vi "FOCUS_V42_H37.vi"(9 "X-pixels":sgl=256.0, 11 "Run":bool) -> (0 "Retrace pixels":sgl, 10 "Pixel Clock (Hz)":sgl)   [LabVIEW 2010] (continued)
                            n2198 = To Unsigned Byte Integer(number=w3929) -> (unsigned 8bit integer=w3921:u8[])
                            n2199 = Add(x=w3896, y=w3900) -> (x+y=w3905:sgl[])
                            n2200 = To Unsigned Byte Integer(number=w3905) -> (unsigned 8bit integer=w3893:u8[])
                          }
                        }
                      }
                    }
                    n2201 = case shown="True" "Overlay Images" {
                      tunnel: w3666 -> [w4140 w4159]
                      tunnel: [w4140 w4142] -> w3813
                      tunnel: w3665 -> [w4139 w4161]
                      tunnel: [w4139 _] -> w3814
                      frame False {
                      }
                      frame True {
                        n2202 = To Word Integer(number=w4159) -> (16bit integer=w4160:i16[])
                        n2203 = Subtract(x=w4160, y=w4161) -> (x-y=w4141:i16[])
                        n2204 = Add(x=w4160, y=w4161) -> (x+y=w4155:i16[])
                        n2205 = Increment(x=w4155) -> (x+1=w4165:i16[])
                        n2206 = Divide(x=w4141, y=w4165) -> (x/y=w4164:dbl[])
                        n2207 = Absolute Value(x=w4141) -> (abs(x)=w4157:i16[])
                        n2208 = Multiply(x=w4164, y=u8 2) -> (x*y=w4162:dbl[])
                        n2209 = Round To Nearest(number=w4162) -> (nearest integer value=w4148:dbl[])
                        n2210 = Divide(x=w4157, y=2.0) -> (x/y=w4154:dbl[])
                        n2211 = Divide(x=w4155, y=2.0) -> (x/y=w4153:dbl[])
                        n2212 = Add(x=w4154, y=w4153) -> (x+y=w4151:dbl[])
                        n2213 = Divide(x=w4151, y=5.0) -> (x/y=w4150:dbl[])
                        n2214 = Round To Nearest(number=w4150) -> (nearest integer value=w4149:dbl[])
                        n2215 = Multiply(x=5.0 ("y"), y=w4149) -> (x*y=w4147:dbl[])
                        n2216 = Add(x=w4148, y=w4147) -> (x+y=w4146:dbl[])
                        n2217 = Subtract(x=w4146, y=2.0) -> (x-y=w4143:dbl[])
                        n2218 = To Unsigned Byte Integer(number=w4143) -> (unsigned 8bit integer=w4142:u8[])
                      }
                    }
                    n2219 = Greater Or Equal?(x=w3724, y=w3723) -> (x >= y?=w3658:bool)
                    n2220 = Sign(1:w3762) -> (0:w3761:i32)
                    n2221 = local write "Scan Backlock"(w3712) -> ()
                    n2222 = case shown="-1" w3761 {
                      tunnel: "Zoom" -> [_ w3966 w3971]
                      frame 0, Default {
                      }
                      frame 1 {
                        n2223 = Multiply(x=w3966, y=sgl 1.25) -> (x*y=w3964:sgl)
                        n2224 = local write "Zoom"(w3964) -> ()
                      }
                      frame -1 {
                        n2225 = Multiply(x=w3971, y=sgl 0.8) -> (x*y=w3967:sgl)
                        n2226 = Greater Or Equal?(x=w3967, y=sgl 0.28) -> (x >= y?=w3969:bool)
                        n2227 = case shown="True" w3969 {
                          tunnel: w3967 -> [_ w3972]
                          frame False {
                          }
                          frame True {
                            n2228 = local write "Zoom"(w3972) -> ()
                          }
                        }
                      }
                    }
                    n2229 = Not(x=w3681) -> (.not. x?=→"On?":bool)
                    n2230 = case shown="True" w3658 {
                      tunnel: w3770 -> [w3976 w4005]
                      tunnel: [w3976 w4004] -> w3769
                      tunnel: w3768 -> [w3977 w3983]
                      tunnel: [w3977 w3991] -> w3767
                      tunnel: w3719 -> [w3974 w3988]
                      tunnel: w3720 -> [w3975 w3985]
                      tunnel: [w3975 w3986] -> w3722
                      tunnel: [w3974 w3989] -> w3721
                      tunnel: [w3973 w3982] -> w3718
                      tunnel: w3717 -> [w3973 w3981]
                      tunnel: "scattering length [µm]" -> [_ w3978]
                      frame False {
                      }
                      frame True {
                        n2231 = local read "Sutter scale z"() -> (w3979:sgl)
                        n2232 = call "VISA MP-285 Get Z Position.vi"("Input: Duty Cluster"=w4005) -> ("Output: Z axis (microns)"=w4003:sgl, "Output: Duty Cluster"=w4004:T18, "error?"=w3982:bool)
                        n2233 = Multiply(x=w3979, y=w4003) -> (x*y=w3991:sgl)
                        n2234 = Equal?(x=TRUE, y="GetFirst") -> (x = y?=w3995:bool)
                        n2235 = Not Equal?(x="GetFirst", y=w3985) -> (x != y?=w3994:bool)
                        n2236 = Equal?(x=TRUE, y="GetLast") -> (x = y?=w3997:bool)
                        n2237 = Not Equal?(x="GetLast", y=w3988) -> (x != y?=w3999:bool)
                        n2238 = Subtract(x=w3991, y=w3983) -> (x-y=w4000:sgl)
                        n2239 = And(x=w3982, y=w3981) -> (x .and. y?=w3980:bool)
                        n2240 = Not Equal To 0?(x=w4000) -> (x != 0?=w4002:bool)
                        n2241 = Compound Arithmetic op=AND(w3995, w3994, w3980) -> (w3993:bool)
                        n2242 = Compound Arithmetic op=AND(w3980, w3997, w3999) -> (w3992:bool)
                        n2243 = Compound Arithmetic op=AND("IntensityAutomatic", w4002, w3980) -> (w3984:bool)
                        n2244 = case shown="True" w3993 {
                          tunnel: w3991 -> [_ w4008]
                          tunnel: "GetFirst" -> [_ w4007]
                          tunnel: [w4006 w4007] -> w3986
                          tunnel: w3985 -> [w4006 _]
                          frame False {
                          }
                          frame True {
                            "FirstPosition" <- w4008
                          }
                        }
                        n2245 = case shown="True" w3992 {
                          tunnel: w3991 -> [_ w4011]
                          tunnel: "GetLast" -> [_ w4010]
                          tunnel: [w4009 w4010] -> w3989
                          tunnel: w3988 -> [w4009 _]
                          frame False {
                          }
                          frame True {
                            "LastPosition" <- w4011
                          }
                        }
                        n2246 = case shown="True" w3984 {
                          tunnel: w4000 -> [_ w4015]
                          tunnel: w3991 -> [_ w4014]
                          tunnel: [w4012 w4014] -> _
                          tunnel: w3983 -> [w4012 _]
                          tunnel: w3978 -> [_ w4013]
                          frame False {
                          }
                          frame True {
                            n2247 = Divide(x=w4015, y=w4013) -> (x/y=w4022:sgl)
                            n2248 = local read "Intensity"() -> (w4020:sgl)
                            n2249 = Exponential(1:w4022) -> (0:w4021:sgl)
                            n2250 = local read "IntensityScaleMax"() -> (w4016:sgl)
                            n2251 = Multiply(x=w4020, y=w4021) -> (x*y=w4018:sgl)
                            n2252 = In Range and Coerce(upper limit=sgl 0.0, x=w4018, lower limit=w4016) -> (coerced(x)=w4017:sgl)  [unwired: 1 out]
                            n2253 = local write "Intensity"(w4017) -> ()
                          }
                        }
                      }
                    }
                    n2254 = Greater Or Equal?(x=w3812, y="Image Update [ms]") -> (x >= y?=w3810:bool)
                    n2255 = Greater Or Equal?(x=w3726, y=w3723) -> (x >= y?=w3654:bool)
                    n2256 = Replace Array Subset(array=w3771, new element=w3813, index (col)=w3726) -> (w3808:u8[][])  [unwired: 1 in]
                    n2257 = Replace Array Subset(array=w3778, new element=w3814, index (col)=w3726) -> (w3807:u8[][])  [unwired: 1 in]
                    n2258 = case shown="True" w3810 {
                      tunnel: [w4135 w4138] -> w3809
                      tunnel: w3795 -> [w4135 _]
                      tunnel: w3808 -> [_ w4137]
                      tunnel: w3807 -> [_ w4136]
                      frame False {
                      }
                      frame True {
                        n2259 = local write "Image 1"(w4137) -> ()
                        n2260 = local write "Image 2"(w4136) -> ()
                        n2261 = Tick Count (ms)() -> (millisecond timer value=w4138:u32)
                      }
                    }
                    n2262 = Unbundle By Name(w3743) -> ("status"=w3738:bool)
                    n2263 = case shown="False" w3654 {
                      tunnel: [w4038 i16 0] -> w3800
                      tunnel: w3726 -> [w4039 _]
                      frame False {
                        n2264 = Increment(x=w4039) -> (x+1=w4038:i16)
                      }
                      frame True {
                      }
                    }
                    n2265 = Unbundle By Name(w3742) -> ("status"=w3673:bool)
                    n2266 = case shown="False" w3658 {
                      tunnel: [w3957 i16 0] -> w3725
                      tunnel: w3724 -> [w3958 _]
                      frame False {
                        n2267 = Increment(x=w3958) -> (x+1=w3957:i16)
                      }
                      frame True {
                      }
                    }
                    n2268 = case shown="True" w3655 {
                      tunnel: w3666 -> [w3820 w3823]
                      tunnel: w3665 -> [w3817 w3822]
                      tunnel: w3664 -> [w3819 _]
                      tunnel: [w3818 w3821] -> w3661
                      frame True {
                        n2269 = Interleave 1D Arrays(w3817, w3820, w3819) -> (w3818:u8[])
                      }
                      frame False {
                        n2270 = Interleave 1D Arrays(w3823, w3822) -> (w3821:u8[])
                      }
                    }
                    n2271 = case shown="True" w3654 {
                      tunnel: w3663 -> [w3833 w3841]
                      tunnel: w3662 -> [w3832 w3840]
                      tunnel: w3661 -> [w3831 w3839]
                      tunnel: [w3830 w3838] -> w3660
                      tunnel: [w3829 w3837] -> w3659
                      frame True {
                        n2272 = Set File Position(offset (in bytes) (0)=768 ("pos offset (0)"), refnum=w3833, from (0:start)=enum16{"start", "end", "current"}."start" ("pos mode (0:2)"), error in=w3832) -> (refnum out=w3826:refnum<file>, error out=w3825:errorcluster)
                        n2273 = Write to Binary File(file (use dialog)=w3826, data=w3831, error in=w3825, 5:FALSE ("prepend array or string size? (T)")) -> (refnum out=w3830:refnum<file>, error out=w3829:errorcluster)  [unwired: 2 in, 1 out]
                      }
                      frame False {
                        n2274 = Set File Position(refnum=w3841, from (0:start)=enum16{"start", "end", "current"}."current" ("pos mode (0:2)"), error in=w3840) -> (refnum out=w3836:refnum<file>, error out=w3835:errorcluster)  [unwired: 1 in]
                        n2275 = Write to Binary File(file (use dialog)=w3836, data=w3839, error in=w3835, 5:FALSE ("prepend array or string size? (T)")) -> (refnum out=w3838:refnum<file>, error out=w3837:errorcluster)  [unwired: 2 in, 1 out]
                      }
                    }
                    n2276 = Unbundle By Name(w3713) -> ("status"=w3737:bool)
                    n2277 = local read "End experiment"() -> (w3733:bool)
                    n2278 = Unbundle By Name(w3739) -> ("status"=w3734:bool)
                    n2279 = Unbundle By Name(w3740) -> ("status"=w3735:bool)
                    n2280 = Unbundle By Name(w3741) -> ("status"=w3736:bool)
                    n2281 = Compound Arithmetic op=OR("stop 2", w3733, w3734, w3735, w3736, w3737, w3738, w3673) -> (w3731:bool)
                  }
                  n2282 = Not Equal?(x=w3575, y=w3574) -> (x != y?=→"IntDevUsed":bool)
                  n2283 = Close File(refnum=w3525, error in=w3524) -> ()  [unwired: 2 out]
                  n2284 = Unbundle(w3622) -> (w3600:sgl, w3599:sgl, w3598:sgl, "Zoom"=w3597:sgl, "x jog"=w3596:sgl, "y jog"=w3595:sgl, w3605:sgl, w3593:sgl)  [unwired: 5 out]
                  n2285 = call-poly <vilib>:"closeMouse.vi"("error in (no error)"=w3586, "device ID"=w3585) -> ("error out"=w3584:errorcluster)  [unwired: 8 in]
                  n2286 = call-poly <vilib>:"closeKeyboard.vi"("error in (no error)"=w3554, "device ID"=w3555) -> ("error out"=w3556:errorcluster)  [unwired: 8 in]
                  n2287 = call <vilib>:"Simple Error Handler.vi"("error in (no error)"=w3584) -> ()  [unwired: 4 in, 5 out]
                  n2288 = call <vilib>:"Simple Error Handler.vi"("error in (no error)"=w3556) -> ()  [unwired: 4 in, 5 out]
                  n2289 = local write "Zoom"(w3597) -> ()
                  n2290 = local write "x jog"(w3596) -> ()
                  n2291 = local write "y jog"(w3595) -> ()
                  n2292 = Multiply(x=w3605, y=sgl -1.0) -> (x*y=w3607:sgl)
                  n2293 = Subtract(x=w3607, y=sgl 360.0) -> (x-y=w3594:sgl)
                  n2294 = local write "Rotation"(w3594) -> ()
                  n2295 = flat-sequence {
                    tunnel: w3614 -> [w3652]
                    tunnel: [w3652] -> w3613
                    tunnel: w3579 -> [w3651]
                    frame #0 {
                      n2296 = Tick Count (ms)() -> (millisecond timer value=w3653:u32)
                      n2297 = local write "Parameters"(w3651) -> ()
                      n2298 = local write "stop"(w3653) -> ()
                    }
                  }
                  n2299 = Bundle(w3600, w3599, w3598, "Zoom"=w3597, "x jog"=w3596, "y jog"=w3595, w3594, w3593) -> (→"Scan Parameters":T32)  [unwired: 1 in]
                }
                frame 1 {
                  # "Iinner while loop runs for n loops, where n = number of averages.\nAll data acquired in this loop enters the average.\nThe z-step is activated each time this loop completes..\nThe outer while loop iterates m times, where m is total number of frames.\nControls are reset after the outer while loop completes.\nThe shutter is closed before and opened after each z-step."
                  # "Frame scan"
                  n2300 = flat-sequence {
                    tunnel: w4241 -> [w4250]
                    tunnel: [w4250] -> w4240
                    frame #0 {
                      n2301 = Tick Count (ms)() -> (millisecond timer value=→"start":u32)
                    }
                  }
                  n2302 = property on="Property Node" class="VI"() -> ("VI Path"=w4201:path)  [unwired: 2 in, 2 out]
                  n2303 = local read "x-step (um)"() -> (w4175:sgl)
                  n2304 = local read "y-step (um)"() -> (w4174:sgl)
                  n2305 = local read "z-step (um)"() -> (w4208:sgl)
                  n2306 = local read "z-positionstart (um)"() -> (w4176:sgl)
                  n2307 = Strip Path(path=w4201) -> (stripped path=w4200:path)  [unwired: 1 out]
                  n2308 = Equal To 0?(x=w4208) -> (x = 0?=w4171:bool)
                  n2309 = Equal To 0?(x=w4175) -> (x = 0?=w4172:bool)
                  n2310 = Equal To 0?(x=w4174) -> (x = 0?=w4173:bool)
                  n2311 = Initialize Array(u8 0 ("element"), w4219, w4218) -> (w4236:u8[][])
                  n2312 = Compound Arithmetic op=AND(w4172, w4173, w4171) -> (w4170:bool)
                  n2313 = Build Path(base path=w4200, name or relative path="Stack.tmp") -> (appended path=w4199:path)
                  n2314 = local write "FirstPosition"(w4176) -> ()
                  n2315 = call <vilib>:"Open_Create_Replace File.vi"("advisory dialog? (display:T)"=FALSE, "function (open:0)"=T8."create or replace", "file path"=w4199) -> ("error out"=w4192:errorcluster, "refnum"=w4194:refnum<file>)  [unwired: 5 in, 2 out]
                  n2316 = Set File Position(refnum=w4194, from (0:start)=enum16{"start", "end", "current"}."start" ("pos mode (rel. to end:1)"), error in=w4192) -> (refnum out=w4168:refnum<file>, error out=w4167:errorcluster)  [unwired: 1 in]
                  n2317 = Write to Binary File(file (use dialog)=w4168, data=w4190, error in=w4167, 5:FALSE ("prepend array or string size? (T)")) -> (refnum out=w4193:refnum<file>, error out=w4191:errorcluster)  [unwired: 2 in, 1 out]
                  n2318 = property on="Property Node" class="VI"() -> ("VI Path"=w4186:path)  [unwired: 2 in, 2 out]
                  n2319 = Strip Path(path=w4186) -> (stripped path=w4185:path)  [unwired: 1 out]
                  n2320 = Build Path(base path=w4185, name or relative path="EEG.tmp") -> (appended path=w4184:path)
                  n2321 = call <vilib>:"Open_Create_Replace File.vi"("advisory dialog? (display:T)"=FALSE, "function (open:0)"=T8."create or replace", "file path"=w4184) -> ("error out"=w4181:errorcluster, "refnum"=w4182:refnum<file>)  [unwired: 5 in, 2 out]
                  n2322 = while {
                    tunnel: [w4337] -> w4247
                    tunnel: [w4336] -> w4239
                    tunnel: w4246 -> [w4335]
                    tunnel: w4240 -> [w4334]
                    tunnel: w4245 -> [w4333]
                    tunnel: w4220 -> [w4259]
                    shift-right: [w4328] -> w4207
                    shift-left: w4236 -> [w4329]
                    shift-right: [w4326] -> w4206
                    shift-left: w4236 -> [w4327]
                    tunnel: [w4296] -> w4233
                    tunnel: w4235 -> [w4287]
                    tunnel: [w4294] -> w4232
                    tunnel: w4234 -> [w4288]
                    tunnel: w4177 -> [w4325]
                    tunnel: [w4324] -> w4221
                    tunnel: w4228 -> [w4323]
                    tunnel: w4226 -> [w4322]
                    tunnel: [w4321] -> w4227
                    tunnel: [w4320] -> w4225
                    tunnel: w4224 -> [w4293]
                    tunnel: w4223 -> [w4292]
                    tunnel: [w4318] -> w4213
                    tunnel: [w4317] -> w4222
                    tunnel: w4217 -> [w4311]
                    tunnel: w4216 -> [w4307]
                    tunnel: [w4310] -> w4215
                    tunnel: [w4309] -> w4214
                    tunnel: [w4285] -> w4212
                    tunnel: [w4299] -> w4210
                    tunnel: w4170 -> [w4272]
                    shift-right: [w4278] -> w4197
                    shift-left: w4193 -> [w4280]
                    shift-right: [w4277] -> w4196
                    shift-left: w4191 -> [w4279]
                    tunnel: w4189 -> [w4270]
                    shift-right: [w4267] -> w4180
                    shift-left: w4182 -> [w4269]
                    shift-right: [w4266] -> w4179
                    shift-left: w4181 -> [w4268]
                    tunnel: w4178 -> [w4265]
                    tunnel: w4169 -> [w4257]
                    i -> [w4285]
                    stop <- w4261 stop-if-true
                    w4273 = 0
                    n2323 = Equal To 0?(x=w4285) -> (x = 0?=w4312:bool)
                    n2324 = Greater Or Equal?(x=w4257, y=u16 3) -> (x >= y?=w4255:bool)
                    n2325 = Tick Count (ms)() -> (millisecond timer value=w4332:u32)
                    n2326 = Equal To 0?(x=w4285) -> (x = 0?=w4283:bool)
                    n2327 = Or(x=w4283, y=w4272) -> (x .or. y?=w4282:bool)
                    n2328 = case shown="False" w4282 {
                      tunnel: w4293 -> [w4348 w4357]
                      tunnel: [w4341 w4357] -> w4291
                      tunnel: w4292 -> [w4347 w4358]
                      tunnel: [w4340 w4358] -> w4290
                      tunnel: w4287 -> [w4345 w4355]
                      tunnel: w4288 -> [w4344 w4356]
                      tunnel: [w4339 w4356] -> w4289
                      tunnel: [w4338 w4355] -> w4286
                      frame False {
                        w4346 = TRUE ("data")
                        n2329 = local write "Shutter open"(w4346) -> ()
                        n2330 = call-poly <vilib>:"DAQmx Write (Digital Bool 1Line 1Point).vi"("task/channels in"=w4348, "data"=w4346, "error in"=w4347) -> ("task out"=w4343:refnum<k21>, "error out"=w4342:errorcluster)  [unwired: 10 in, 1 out]
                        n2331 = flat-sequence {
                          tunnel: w4345 -> [w4354]
                          tunnel: w4344 -> [w4353]
                          tunnel: w4343 -> [w4352]
                          tunnel: [w4352] -> w4341
                          tunnel: [w4351] -> w4340
                          tunnel: w4342 -> [w4351]
                          tunnel: [w4350] -> w4339
                          tunnel: [w4349] -> w4338
                          frame #0 {
                            n2332 = call <vilib>:"DAQmx Start Task.vi"("task/channels in"=w4354, "error in"=w4353) -> ("task out"=w4349:refnum<k21>, "error out"=w4350:errorcluster)  [unwired: 12 in]
                          }
                        }
                      }
                      frame True {
                      }
                    }
                    n2333 = Unbundle By Name(w4292) -> ("status"=w4306:bool)
                    n2334 = Unbundle By Name(w4307) -> ("status"=w4305:bool)
                    n2335 = Increment(x=w4285) -> (x+1=w4319:i32)
                    "#" <- w4319
                    n2336 = Compound Arithmetic op=OR(w4306, w4305) -> (w4304:bool)
                    n2337 = while {
                      tunnel: [w4487] -> w4337
                      tunnel: [w4489] -> w4336
                      tunnel: w4335 -> [w4511]
                      tunnel: w4334 -> [w4510]
                      shift-right: [w4517] -> w4276
                      shift-left: w4259 -> [w4516]
                      tunnel: w4333 -> [w4475]
                      shift-right: [w4518] -> w4275
                      shift-left: w4259 -> [w4519]
                      tunnel: [w4499] -> w4301
                      tunnel: [w4500] -> w4302
                      tunnel: ["z-step (um)"] -> w4284
                      tunnel: ["y-step (um)"] -> w4330
                      tunnel: ["x-step (um)"] -> w4331
                      shift-right: [w4532] -> _
                      shift-left: w4332 -> [w4533]
                      tunnel: w4312 -> [w4514]
                      tunnel: [w4458] -> w4297
                      tunnel: w4286 -> [w4458]
                      tunnel: [w4457] -> w4295
                      tunnel: w4289 -> [w4457]
                      tunnel: w4323 -> [w4513]
                      tunnel: w4322 -> [w4512]
                      tunnel: [w4506] -> w4321
                      tunnel: [w4477] -> w4320
                      tunnel: w4304 -> [w4498]
                      tunnel: [w4496] -> w4300
                      shift-right: [w4483] -> _
                      shift-left: w4273 -> [w4436]
                      shift-right: [w4482] -> _
                      shift-left: w4273 -> [w4435]
                      tunnel: w4270 -> [w4481]
                      shift-right: [w4468] -> w4267
                      shift-left: w4269 -> [w4471]
                      shift-right: [w4467] -> w4266
                      shift-left: w4268 -> [w4470]
                      tunnel: w4265 -> [w4452]
                      tunnel: w4257 -> [w4443]
                      shift-right: [w4434] -> w4258
                      shift-left: w4259 -> [w4437]
                      i -> [w4451]
                      stop <- w4497 stop-if-true
                      n2338 = local read "Scan Cut-Off (either end)"() -> (w4480:sgl)
                      n2339 = Equal To 0?(x="z-step (um)") -> (x = 0?=w4446:bool)
                      n2340 = Equal To 0?(x="y-step (um)") -> (x = 0?=w4447:bool)
                      n2341 = Equal To 0?(x="x-step (um)") -> (x = 0?=w4448:bool)
                      n2342 = Equal To 0?(x=w4451) -> (x = 0?=w4495:bool)
                      n2343 = call-poly <vilib>:"DAQmx Read (Analog 2D DBL NChan NSamp).vi"("task/channels in"=w4513, "number of samples per channel"=w4475, "error in"=w4512) -> ("task out"=w4506:refnum<k21>, "data"=w4476:dbl[][], "error out"=w4477:errorcluster)  [unwired: 10 in]
                      n2344 = Compound Arithmetic op=AND(w4446, w4447, w4448) -> (w4445:bool)
                      n2345 = local read "End experiment"() -> (w4500:bool)
                      n2346 = local read "Cusp Delay"() -> (w4478:sgl)
                      n2347 = case shown="True" w4445 {
                        tunnel: w4514 -> [_ w4641]
                        tunnel: w4495 -> [w4638 w4640]
                        tunnel: [w4638 w4639] -> w4494
                        frame False {
                        }
                        frame True {
                          n2348 = And(x=w4640, y=w4641) -> (x .and. y?=w4639:bool)
                        }
                      }
                      n2349 = case shown="False" w4494 {
                        tunnel: w4475 -> [w4642 w4648]
                        tunnel: [w4642 w4644] -> w4459
                        tunnel: w4480 -> [w4643 w4647]
                        tunnel: [w4643 w4646] -> w4504
                        tunnel: w4481 -> [_ w4645]
                        frame False {
                        }
                        frame True {
                          n2350 = Add(x=w4648, y=w4645) -> (x+y=w4644:sgl)
                          n2351 = Add(x=w4647, y=w4645) -> (x+y=w4646:sgl)
                        }
                      }
                      n2352 = call-poly <vilib>:"DAQmx Read (Digital 1D U32 1Chan NSamp).vi"("task/channels in"=w4511, "number of samples per channel"=w4459, "error in"=w4510) -> ("task out"=w4488:refnum<k21>, "data"=w4462:u32[], "error out"=w4490:errorcluster)  [unwired: 10 in]
                      n2353 = local read "X-pixels"() -> (w4509:sgl)
                      n2354 = local read "Overlay Images"() -> (w4515:bool)
                      n2355 = local read "stop 2"() -> (w4499:bool)
                      n2356 = Unbundle By Name(w4490) -> ("status"=w4502:bool)
                      n2357 = Unbundle By Name(w4457) -> ("status"=w4503:bool)
                      n2358 = Add(x=w4504, y=w4478) -> (x+y=w4479:sgl)
                      n2359 = local read "total y pixels"() -> (w4463:sgl)
                      n2360 = case shown="1" w4452 {
                        tunnel: w4451 -> [_ w4626]
                        tunnel: w4462 -> [w4621 w4624]
                        tunnel: [w4621 w4623] -> w4460
                        frame 0, Default {
                        }
                        frame 1 {
                          n2361 = local read "Shift"() -> (w4622:sgl)
                          n2362 = call "testoddevenFOCUS.vi"("Numeric"=w4626) -> ("Boolean"=w4625:bool)
                          n2363 = case shown="True" w4625 {
                            tunnel: w4624 -> [w4628 w4631]
                            tunnel: [w4627 w4629] -> w4623
                            tunnel: w4622 -> [_ w4630]
                            frame False {
                              n2364 = Reverse 1D Array(array=w4628) -> (reversed array=w4627:u32[])
                            }
                            frame True {
                              n2365 = Rotate 1D Array(1:w4631, 2:w4630) -> (0:w4629:u32[])
                            }
                          }
                        }
                      }
                      n2366 = Array Subset "Extract DI0"(array=w4460, index=w4479, length=w4509) -> (w4461:u32[])
                      n2367 = Split Number(x=w4461) -> (hi(x)=w4507:u16[], lo(x)=w4444:u16[])
                      n2368 = property class="DAQmx Read"(reference=w4488, error in=w4490) -> (reference out=w4487:refnum<k21>, error out=w4489:errorcluster, "Status:Available Samples Per Channel"=w4486:u32)
                      n2369 = case shown="0, Default" w4443 {
                        tunnel: w4507 -> [w4543 w4548 w4553 w4558 w4563 w4568]
                        tunnel: [w4542 w4547 w4550 w4557 w4562 w4565] -> w4456
                        tunnel: [w4540 w4545 w4552 w4555 w4560 w4567] -> w4454
                        tunnel: w4444 -> [w4541 w4546 w4551 w4556 w4561 w4566]
                        tunnel: [w4539 w4544 w4549 w4554 w4559 w4564] -> w4433
                        frame 0, Default {
                          n2370 = Split Number(x=w4543) -> (hi(x)=w4542:u8[], lo(x)=w4540:u8[])
                          n2371 = Split Number(x=w4541) -> (lo(x)=w4539:u8[])  [unwired: 1 out]
                        }
                        frame 1 {
                          n2372 = Split Number(x=w4548) -> (hi(x)=w4547:u8[], lo(x)=w4544:u8[])
                          n2373 = Split Number(x=w4546) -> (lo(x)=w4545:u8[])  [unwired: 1 out]
                        }
                        frame 2 {
                          n2374 = Split Number(x=w4553) -> (hi(x)=w4549:u8[], lo(x)=w4552:u8[])
                          n2375 = Split Number(x=w4551) -> (lo(x)=w4550:u8[])  [unwired: 1 out]
                        }
                        frame 3 {
                          n2376 = Split Number(x=w4558) -> (hi(x)=w4557:u8[], lo(x)=w4555:u8[])
                          n2377 = Split Number(x=w4556) -> (lo(x)=w4554:u8[])  [unwired: 1 out]
                        }
                        frame 4 {
                          n2378 = Split Number(x=w4563) -> (hi(x)=w4562:u8[], lo(x)=w4559:u8[])
                          n2379 = Split Number(x=w4561) -> (lo(x)=w4560:u8[])  [unwired: 1 out]
                        }
                        frame 5 {
                          n2380 = Split Number(x=w4568) -> (hi(x)=w4564:u8[], lo(x)=w4567:u8[])
                          n2381 = Split Number(x=w4566) -> (lo(x)=w4565:u8[])  [unwired: 1 out]
                        }
                      }
                      n2382 = Multiply(x="Averaging", y=w4463) -> (x*y=w4536:sgl)
                      n2383 = Increment(x=w4451) -> (x+1=w4508:i32)
                      n2384 = Equal?(x=w4508, y=w4536) -> (x = y?=w4501:bool)
                      n2385 = Compound Arithmetic op=OR(w4503, w4502) -> (w4496:bool)
                      n2386 = Transpose 2D Array(2D array=w4476) -> (transposed array=w4469:dbl[][])
                      n2387 = Divide(x=w4508, y=w4463) -> (x/y=w4465:sgl)
                      n2388 = local write "Scan Backlock"(w4486) -> ()
                      n2389 = Round Toward +Infinity(x=w4465) -> (ceil(x): smallest int >= x=w4464:sgl)
                      "#" <- w4464
                      n2390 = case shown="1" w4452 {
                        tunnel: w4456 -> [w4571 w4578]
                        tunnel: [w4571 w4577] -> w4455
                        tunnel: w4451 -> [_ w4580]
                        tunnel: w4454 -> [w4570 w4575]
                        tunnel: [w4570 w4574] -> w4453
                        tunnel: w4433 -> [w4569 w4573]
                        tunnel: [w4569 w4572] -> w4432
                        frame 0, Default {
                        }
                        frame 1 {
                          n2391 = local read "Shift"() -> (w4576:sgl)
                          n2392 = call "testoddevenFOCUS.vi"("Numeric"=w4580) -> ("Boolean"=w4579:bool)
                          n2393 = case shown="True" w4579 {
                            tunnel: w4578 -> [w4583 w4610]
                            tunnel: [w4583 w4612] -> w4577
                            tunnel: w4576 -> [_ w4586]
                            tunnel: w4575 -> [w4582 w4598]
                            tunnel: [w4582 w4597] -> w4574
                            tunnel: w4573 -> [w4581 w4585]
                            tunnel: [w4581 w4584] -> w4572
                            frame False {
                            }
                            frame True {
                              n2394 = Round Toward -Infinity(1:w4586) -> (0:w4602:sgl)
                              n2395 = Round Toward -Infinity(1:w4586) -> (0:w4617:sgl)
                              n2396 = Round Toward -Infinity(1:w4586) -> (0:w4593:sgl)
                              n2397 = To Word Integer(number=w4598) -> (16bit integer=w4608:i16[])
                              n2398 = To Word Integer(number=w4610) -> (16bit integer=w4609:i16[])
                              n2399 = To Word Integer(number=w4585) -> (16bit integer=w4587:i16[])
                              n2400 = Array Subset(array=w4608, index=1) -> (w4601:i16[])  [unwired: 1 in]
                              n2401 = Array Subset(array=w4609, index=1) -> (w4618:i16[])  [unwired: 1 in]
                              n2402 = Array Subset(array=w4587, index=1) -> (w4594:i16[])  [unwired: 1 in]
                              n2403 = Subtract(x=w4586, y=w4602) -> (x-y=w4603:sgl)
                              n2404 = Subtract(x=w4586, y=w4617) -> (x-y=w4616:sgl)
                              n2405 = Subtract(x=w4586, y=w4593) -> (x-y=w4592:sgl)
                              n2406 = Subtract(x=w4608, y=w4601) -> (x-y=w4605:i16[])
                              n2407 = Subtract(x=w4609, y=w4618) -> (x-y=w4614:i16[])
                              n2408 = Subtract(x=w4587, y=w4594) -> (x-y=w4590:i16[])
                              n2409 = Build Array (concatenate)(0 ("index"), w4605) -> (w4606:i32[])
                              n2410 = Build Array (concatenate)(0 ("index"), w4614) -> (w4613:i32[])
                              n2411 = Build Array (concatenate)(0 ("index"), w4590) -> (w4589:i32[])
                              n2412 = Multiply(x=w4603, y=w4606) -> (x*y=w4604:sgl[])
                              n2413 = Multiply(x=w4616, y=w4613) -> (x*y=w4615:sgl[])
                              n2414 = Multiply(x=w4592, y=w4589) -> (x*y=w4591:sgl[])
                              n2415 = Add(x=w4608, y=w4604) -> (x+y=w4599:sgl[])
                              n2416 = To Unsigned Byte Integer(number=w4599) -> (unsigned 8bit integer=w4597:u8[])
                              n2417 = Add(x=w4609, y=w4615) -> (x+y=w4620:sgl[])
                              n2418 = To Unsigned Byte Integer(number=w4620) -> (unsigned 8bit integer=w4612:u8[])
                              n2419 = Add(x=w4587, y=w4591) -> (x+y=w4596:sgl[])
                              n2420 = To Unsigned Byte Integer(number=w4596) -> (unsigned 8bit integer=w4584:u8[])
                            }
                          }
                        }
                      }
                      n2421 = case shown="True" w4515 {
                        tunnel: w4455 -> [w4654 w4657]
                        tunnel: [w4654 w4655] -> w4521
                        tunnel: w4453 -> [w4653 w4656]
                        tunnel: [w4653 _] -> w4520
                        frame False {
                        }
                        frame True {
                          n2422 = To Word Integer(number=w4657) -> (16bit integer=w4662:i16[])
                          n2423 = Subtract(x=w4662, y=w4656) -> (x-y=w4663:i16[])
                          n2424 = Add(x=w4662, y=w4656) -> (x+y=w4667:i16[])
                          n2425 = Increment(x=w4667) -> (x+1=w4658:i16[])
                          n2426 = Divide(x=w4663, y=w4658) -> (x/y=w4659:dbl[])
                          n2427 = Absolute Value(x=w4663) -> (abs(x)=w4665:i16[])
                          n2428 = Multiply(x=w4659, y=u8 2) -> (x*y=w4661:dbl[])
                          n2429 = Round To Nearest(number=w4661) -> (nearest integer value=w4674:dbl[])
                          n2430 = Divide(x=w4665, y=2.0) -> (x/y=w4668:dbl[])
                          n2431 = Divide(x=w4667, y=2.0) -> (x/y=w4669:dbl[])
                          n2432 = Add(x=w4668, y=w4669) -> (x+y=w4671:dbl[])
                          n2433 = Divide(x=w4671, y=5.0) -> (x/y=w4672:dbl[])
                          n2434 = Round To Nearest(number=w4672) -> (nearest integer value=w4673:dbl[])
                          n2435 = Multiply(x=5.0 ("y"), y=w4673) -> (x*y=w4675:dbl[])
                          n2436 = Add(x=w4674, y=w4675) -> (x+y=w4676:dbl[])
                          n2437 = Subtract(x=w4676, y=2.0) -> (x-y=w4679:dbl[])
                          n2438 = To Unsigned Byte Integer(number=w4679) -> (unsigned 8bit integer=w4655:u8[])
                        }
                      }
                      n2439 = Compound Arithmetic op=OR(w4496, w4501, w4500, w4499, w4498) -> (w4497:bool)
                      n2440 = Subtract(x=w4465, y=w4464) -> (x-y=w4492:sgl)
                      n2441 = Equal To 0?(x=w4492) -> (x = 0?=w4466:bool)
                      n2442 = Tick Count (ms)() -> (millisecond timer value=w4535:u32)
                      n2443 = local read "total y pixels"() -> (w4538:sgl)
                      n2444 = while {
                        tunnel: w4538 -> [w4682]
                        shift-right: [w4683] -> _
                        shift-left: w4451 -> [w4681]
                        tunnel: [w4681] -> _
                        tunnel: [w4680] -> _
                        i -> [w4680]
                        stop <- w4684 stop-if-true
                        n2445 = Subtract(x=w4681, y=w4682) -> (x-y=w4683:sgl)
                        n2446 = Less?(x=w4681, y=w4682) -> (x < y?=w4684:bool)
                      }
                      n2447 = Decrement(x=w4463) -> (x-1=w4485:sgl)
                      n2448 = Index Array(array=w4469, index (col)=3 ("disabled index (col)")) -> (element=w4474:dbl[])  [unwired: 1 in]
                      n2449 = Subtract(x=w4535, y=w4533) -> (x-y=w4534:u32)
                      n2450 = Set File Position(refnum=w4471, from (0:start)=enum16{"start", "end", "current"}."current" ("pos mode (0:2)"), error in=w4470) -> (refnum out=w4431:refnum<file>, error out=w4430:errorcluster)  [unwired: 1 in]
                      n2451 = Greater Or Equal?(x=w4436, y=w4485) -> (x >= y?=w4484:bool)
                      n2452 = Write to Binary File(file (use dialog)=w4431, data=w4474, error in=w4430, 5:FALSE ("prepend array or string size? (T)")) -> (refnum out=w4468:refnum<file>, error out=w4467:errorcluster)  [unwired: 2 in, 1 out]
                      n2453 = local read "Image Update [ms]"() -> (w4505:u32)
                      n2454 = Index Array(array=w4516, index (col)=w4436) -> (element=w4522:u8[])  [unwired: 1 in]
                      n2455 = case shown="True" w4484 {
                        tunnel: [w4633 i16 0] -> w4483
                        tunnel: w4436 -> [w4634 _]
                        tunnel: w4435 -> [w4632 w4636]
                        tunnel: [w4632 w4635] -> w4482
                        frame False {
                          n2456 = Increment(x=w4634) -> (x+1=w4633:i32)
                        }
                        frame True {
                          n2457 = Increment(x=w4636) -> (x+1=w4635:i32)
                        }
                      }
                      n2458 = Multiply(x=w4522, y=w4435) -> (x*y=w4523:i32[])
                      n2459 = Add(x=w4523, y=w4521) -> (x+y=w4525:i32[])
                      n2460 = Index Array(array=w4519, index (col)=w4436) -> (element=w4531:u8[])  [unwired: 1 in]
                      n2461 = Greater Or Equal?(x=w4534, y=w4505) -> (x >= y?=w4491:bool)
                      n2462 = Increment(x=w4435) -> (x+1=w4524:i32)
                      n2463 = Multiply(x=w4531, y=w4435) -> (x*y=w4530:i32[])
                      n2464 = Divide(x=w4525, y=w4524) -> (x/y=w4526:dbl[])
                      n2465 = Add(x=w4530, y=w4520) -> (x+y=w4528:i32[])
                      n2466 = Increment(x=w4435) -> (x+1=w4529:i32)
                      n2467 = Index Array(array=w4437, index (col)=w4436) -> (element=w4438:u8[])  [unwired: 1 in]
                      n2468 = Replace Array Subset(array=w4516, new element=w4526, index (col)=w4436) -> (w4517:u8[][])  [unwired: 1 in]
                      n2469 = Or(x=w4466, y=w4491) -> ()  [unwired: 1 out]
                      n2470 = Divide(x=w4528, y=w4529) -> (x/y=w4527:dbl[])
                      n2471 = Multiply(x=w4438, y=w4435) -> (x*y=w4439:i32[])
                      n2472 = Add(x=w4439, y=w4432) -> (x+y=w4441:i32[])
                      n2473 = Increment(x=w4435) -> (x+1=w4440:i32)
                      n2474 = Replace Array Subset(array=w4519, new element=w4527, index (col)=w4436) -> (w4518:u8[][])  [unwired: 1 in]
                      n2475 = Divide(x=w4441, y=w4440) -> (x/y=w4442:dbl[])
                      n2476 = case shown="True" w4466 {
                        tunnel: [w4649 w4652] -> w4532
                        tunnel: w4533 -> [w4649 _]
                        tunnel: w4517 -> [_ w4651]
                        tunnel: w4518 -> [_ w4650]
                        frame False {
                        }
                        frame True {
                          n2477 = local write "Image 2"(w4650) -> ()
                          n2478 = local write "Image 1"(w4651) -> ()
                          n2479 = Tick Count (ms)() -> (millisecond timer value=w4652:u32)
                        }
                      }
                      n2480 = Replace Array Subset(array=w4437, new element=w4442, index (col)=w4436) -> (w4434:u8[][])  [unwired: 1 in]
                    }
                    n2481 = Not(x="Go further?") -> (.not. x?=w4264:bool)
                    n2482 = Equal?(x="Number of frames", y=w4319) -> (x = y?=w4303:bool)
                    n2483 = Compound Arithmetic op=OR(w4300, w4301, w4302, w4303, w4304) -> (w4271:bool)
                    n2484 = Or(x=w4271, y=w4272) -> (x .or. y?=w4262:bool)
                    n2485 = Select(t=w4264, s="Go further?", f=w4262) -> (s? t:f=w4260:bool)
                    n2486 = local read "IntensityAutomatic"() -> (w4298:bool)
                    n2487 = case shown="False" w4260 {
                      tunnel: [w4370 w4420] -> w4261
                      tunnel: w4331 -> [w4365 _]
                      tunnel: w4330 -> [w4364 _]
                      tunnel: w4284 -> [w4363 _]
                      tunnel: w4325 -> [w4389 w4428]
                      tunnel: [w4388 w4428] -> w4324
                      tunnel: w4291 -> [w4374 w4425]
                      tunnel: w4290 -> [w4373 w4424]
                      tunnel: [w4372 w4425] -> w4318
                      tunnel: [w4371 w4424] -> w4317
                      tunnel: w4311 -> [w4384 w4427]
                      tunnel: w4307 -> [w4383 w4426]
                      tunnel: [w4382 w4427] -> w4310
                      tunnel: [w4381 w4426] -> w4309
                      tunnel: [w4380 w4423] -> w4299
                      tunnel: w4298 -> [w4379 _]
                      tunnel: w4297 -> [w4377 w4422]
                      tunnel: w4295 -> [w4378 w4421]
                      tunnel: [w4376 w4422] -> w4296
                      tunnel: [w4375 w4421] -> w4294
                      tunnel: w4271 -> [w4370 w4420]
                      frame False {
                        n2488 = local read "Sutter scale x"() -> (w4366:sgl)
                        n2489 = local read "Sutter scale y"() -> (w4367:sgl)
                        n2490 = local read "Sutter scale z"() -> (w4368:sgl)
                        n2491 = case shown="True" w4379 {
                          tunnel: w4384 -> [w4405 w4414]
                          tunnel: w4383 -> [w4404 w4413]
                          tunnel: [w4405 w4412] -> w4382
                          tunnel: [w4404 w4411] -> w4381
                          tunnel: [w4403 w4406] -> w4380
                          tunnel: w4363 -> [_ w4407]
                          frame False {
                            n2492 = local read "Intensity"() -> (w4403:sgl)
                          }
                          frame True {
                            n2493 = local read "scattering length [µm]"() -> (w4417:sgl)
                            n2494 = Divide(x=w4407, y=w4417) -> (x/y=w4419:sgl)
                            n2495 = Exponential(1:w4419) -> (0:w4418:sgl)
                            n2496 = local read "Intensity"() -> (w4416:sgl)
                            n2497 = local read "IntensityScaleMax"() -> (w4408:sgl)
                            n2498 = Multiply(x=w4416, y=w4418) -> (x*y=w4409:sgl)
                            n2499 = In Range and Coerce(upper limit=sgl 0.0, x=w4409, lower limit=w4408) -> (coerced(x)=w4406:sgl)  [unwired: 1 out]
                            n2500 = local write "Intensity"(w4406) -> ()
                            n2501 = Build Array(sgl 0.0 ("element"), w4406) -> ()  [unwired: 1 out]
                            n2502 = call-poly <vilib>:"DAQmx Write (Analog DBL 1Chan 1Samp).vi"("task/channels in"=w4414, "data"=w4406, "error in"=w4413) -> ("task out"=w4412:refnum<k21>, "error out"=w4411:errorcluster)  [unwired: 10 in, 1 out]
                          }
                        }
                        n2503 = Divide(x=w4365, y=w4366) -> (x/y=w4385:sgl)
                        n2504 = Divide(x=w4364, y=w4367) -> (x/y=w4386:sgl)
                        n2505 = Divide(x=w4363, y=w4368) -> (x/y=w4387:sgl)
                        n2506 = Not Equal To 0?(x=w4363) -> (x != 0?=w4361:bool)
                        n2507 = Not Equal To 0?(x=w4364) -> (x != 0?=w4362:bool)
                        n2508 = Not Equal To 0?(x=w4365) -> (x != 0?=w4360:bool)
                        n2509 = call "VISA MP-285 Step.vi"("Input: Duty Cluster"=w4389, "Input: Delta Z axis (microns)"=w4387, "Input: Delta Y axis (microns)"=w4386, "Input: Delta X axis (microns)"=w4385) -> ("Output: Duty Cluster"=w4388:T18)  [unwired: 3 out]
                        n2510 = Wait (ms)(milliseconds to wait=u32 50) -> ()  [unwired: 1 out]
                        n2511 = Compound Arithmetic op=OR(w4361, w4362, w4360) -> (w4359:bool)
                        n2512 = case shown="True" w4359 {
                          tunnel: w4378 -> [w4392 w4402]
                          tunnel: w4377 -> [w4393 w4401]
                          tunnel: [w4393 w4400] -> w4376
                          tunnel: [w4392 w4399] -> w4375
                          tunnel: w4374 -> [w4391 w4398]
                          tunnel: w4373 -> [w4390 w4397]
                          tunnel: [w4391 w4396] -> w4372
                          tunnel: [w4390 w4395] -> w4371
                          frame False {
                          }
                          frame True {
                            w4394 = FALSE ("data")
                            n2513 = call <vilib>:"DAQmx Stop Task.vi"("task/channels in"=w4401, "error in"=w4402) -> ("task out"=w4400:refnum<k21>, "error out"=w4399:errorcluster)  [unwired: 12 in]
                            n2514 = local write "Shutter open"(w4394) -> ()
                            n2515 = call-poly <vilib>:"DAQmx Write (Digital Bool 1Line 1Point).vi"("task/channels in"=w4398, "data"=w4394, "error in"=w4397) -> ("task out"=w4396:refnum<k21>, "error out"=w4395:errorcluster)  [unwired: 10 in, 1 out]
                          }
                        }
                      }
                      frame True {
                        n2516 = local read "Intensity"() -> (w4423:sgl)
                      }
                    }
                    "frame scan finished?" <- w4261
                    n2517 = call "ConvertImagesDataFOCUS.vi"("Save mode"=w4255, "Image3"=w4258, "Image2"=w4275, "Image1"=w4276) -> ("Data"=w4274:u8[])
                    n2518 = Set File Position(refnum=w4280, from (0:start)=enum16{"start", "end", "current"}."current" ("pos mode (0:2)"), error in=w4279) -> (refnum out=w4254:refnum<file>, error out=w4253:errorcluster)  [unwired: 1 in]
                    n2519 = local read "Y-lines"() -> (w4314:sgl)
                    n2520 = Write to Binary File(file (use dialog)=w4254, data=w4274, error in=w4253, 5:FALSE ("prepend array or string size? (T)")) -> (refnum out=w4278:refnum<file>, error out=w4277:errorcluster)  [unwired: 2 in, 1 out]
                    n2521 = Multiply(x=w4314, y=w4285) -> (x*y=w4313:sgl)
                    n2522 = Replace Array Subset(array=w4327, new element=w4275, index (row)=0 ("disabled index (row)"), index (col)=w4313) -> (w4326:u8[][])
                    n2523 = Replace Array Subset(array=w4329, new element=w4276, index (row)=0 ("disabled index (row)"), index (col)=w4313) -> (w4328:u8[][])
                  }
                  n2524 = local read "Intensity"() -> (w4211:sgl)
                  n2525 = Not Equal?(x=w4210, y=w4211) -> (x != y?=w4209:bool)
                  n2526 = local write "IntDevUsed"(w4209) -> ()
                  n2527 = Close File(refnum=w4197, error in=w4196) -> ()  [unwired: 2 out]
                  n2528 = Close File(refnum=w4180, error in=w4179) -> ()  [unwired: 2 out]
                  n2529 = flat-sequence {
                    tunnel: w4239 -> [w4248]
                    tunnel: [w4248] -> w4238
                    frame #0 {
                      n2530 = Tick Count (ms)() -> (millisecond timer value=→"stop":u32)
                    }
                  }
                }
                frame 2 {
                  # "Straight line scan"
                  n2531 = flat-sequence {
                    tunnel: w4734 -> [w4744]
                    tunnel: [w4744] -> w4733
                    frame #0 {
                      n2532 = Tick Count (ms)() -> (millisecond timer value=w4745:u32)
                      n2533 = local write "start"(w4745) -> ()
                    }
                  }
                  n2534 = Decrement(x=w4713) -> (x-1=w4712:sgl)
                  n2535 = Unbundle By Name(w4719) -> ("status"=w4717:bool)
                  n2536 = property on="Image 1" class="IntGraph (strict)"("Y Scale.Range:Maximum"=w4712) -> ()  [unwired: 2 in, 2 out]
                  n2537 = Initialize Array(u8 0 ("element"), w4713, w4714) -> (w4715:u8[][])
                  n2538 = Greater Or Equal?(x=w4690, y=u16 3) -> (x >= y?=w4688:bool)
                  n2539 = property on="Property Node" class="VI"() -> ("VI Path"=w4704:path)  [unwired: 2 in, 2 out]
                  n2540 = Unbundle By Name(w4720) -> ("status"=w4718:bool)
                  n2541 = Tick Count (ms)() -> (millisecond timer value=w4735:u32)
                  n2542 = property on="Image 2" class="IntGraph (strict)"("Y Scale.Range:Maximum"=w4712) -> ()  [unwired: 2 in, 2 out]
                  n2543 = Strip Path(path=w4704) -> (stripped path=w4703:path)  [unwired: 1 out]
                  n2544 = Build Path(base path=w4703, name or relative path="Stack.tmp") -> (appended path=w4702:path)
                  n2545 = call <vilib>:"Open_Create_Replace File.vi"("advisory dialog? (display:T)"=FALSE, "function (open:0)"=T8."create or replace", "file path"=w4702) -> ("error out"=w4695:errorcluster, "refnum"=w4697:refnum<file>)  [unwired: 5 in, 2 out]
                  n2546 = Set File Position(refnum=w4697, from (0:start)=enum16{"start", "end", "current"}."start" ("pos mode (rel. to end:1)"), error in=w4695) -> (refnum out=w4687:refnum<file>, error out=w4686:errorcluster)  [unwired: 1 in]
                  n2547 = Write to Binary File(file (use dialog)=w4687, data=w4693, error in=w4686, 5:FALSE ("prepend array or string size? (T)")) -> (refnum out=w4696:refnum<file>, error out=w4694:errorcluster)  [unwired: 2 in, 1 out]
                  n2548 = while {
                    tunnel: [w4770] -> w4737
                    tunnel: [w4768] -> w4732
                    tunnel: w4738 -> [w4796]
                    tunnel: w4733 -> [w4786]
                    shift-right: [w4815] -> w4711
                    shift-left: w4715 -> [w4817]
                    tunnel: w4739 -> [w4801]
                    shift-right: [w4814] -> w4710
                    shift-left: w4715 -> [w4816]
                    shift-right: [w4808] -> _
                    shift-left: w4735 -> [w4809]
                    tunnel: w4727 -> [w4797]
                    tunnel: w4726 -> [w4787]
                    tunnel: [w4797] -> w4725
                    tunnel: [w4787] -> w4724
                    tunnel: [w4792] -> w4721
                    tunnel: w4718 -> [w4785]
                    tunnel: w4717 -> [w4782]
                    tunnel: w4714 -> [w4777]
                    shift-right: [w4773] -> w4699
                    shift-left: w4696 -> [w4775]
                    shift-right: [w4772] -> w4700
                    shift-left: w4694 -> [w4774]
                    tunnel: w4692 -> [w4766]
                    tunnel: w4691 -> [w4762]
                    tunnel: w4690 -> [w4760]
                    tunnel: w4688 -> [w4751]
                    i -> [w4763]
                    stop <- w4778 stop-if-true
                    n2549 = local read "Scan Cut-Off (either end)"() -> (w4799:sgl)
                    n2550 = Equal To 0?(x=w4763) -> (x = 0?=w4800:bool)
                    n2551 = Unbundle By Name(w4786) -> ("status"=w4783:bool)
                    n2552 = case shown="False" w4800 {
                      tunnel: w4801 -> [w4919 w4924]
                      tunnel: [w4919 w4923] -> w4795
                      tunnel: w4799 -> [w4918 w4922]
                      tunnel: [w4918 w4921] -> w4788
                      tunnel: w4766 -> [_ w4920]
                      frame False {
                      }
                      frame True {
                        n2553 = Add(x=w4924, y=w4920) -> (x+y=w4923:sgl)
                        n2554 = Add(x=w4922, y=w4920) -> (x+y=w4921:sgl)
                      }
                    }
                    n2555 = call-poly <vilib>:"DAQmx Read (Digital 1D U32 1Chan NSamp).vi"("task/channels in"=w4796, "number of samples per channel"=w4795, "error in"=w4786) -> ("task out"=w4771:refnum<k21>, "data"=w4765:u32[], "error out"=w4769:errorcluster)  [unwired: 10 in]
                    n2556 = case shown="1" w4762 {
                      tunnel: w4763 -> [_ w4912]
                      tunnel: w4765 -> [w4907 w4910]
                      tunnel: [w4907 w4909] -> w4764
                      frame 0, Default {
                      }
                      frame 1 {
                        n2557 = local read "Shift"() -> (w4908:sgl)
                        n2558 = call "testoddevenFOCUS.vi"("Numeric"=w4912) -> ("Boolean"=w4911:bool)
                        n2559 = case shown="False" w4911 {
                          tunnel: w4910 -> [w4914 w4917]
                          tunnel: [w4913 w4915] -> w4909
                          tunnel: w4908 -> [_ w4916]
                          frame False {
                            n2560 = Reverse 1D Array(array=w4914) -> (reversed array=w4913:u32[])
                          }
                          frame True {
                            n2561 = Rotate 1D Array(1:w4917, 2:w4916) -> (0:w4915:u32[])
                          }
                        }
                      }
                    }
                    n2562 = local read "Cusp Delay"() -> (w4790:sgl)
                    n2563 = local read "X-pixels"() -> (w4791:sgl)
                    n2564 = Add(x=w4788, y=w4790) -> (x+y=w4789:sgl)
                    n2565 = local read "End experiment"() -> (w4780:bool)
                    n2566 = Unbundle By Name(w4787) -> ("status"=w4784:bool)
